vi "Prune to Directory.vi"(8 "error in (no error)":errorcluster, 11 "Path In":path) -> (0 "error out":errorcluster, 3 "Directory":path)   [LabVIEW 2021, in "File_CIF_U.lvlib"]
doc: "Check if file or directory. If file prune and return the directory."
uses:
  File_CIF_U.lvlib
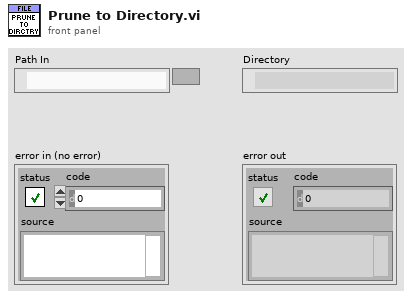
[diagram p1: front panel]
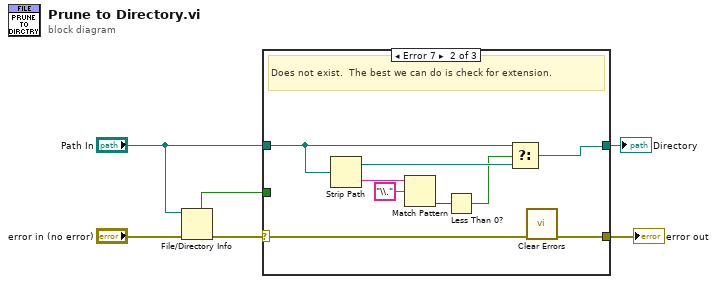
[diagram p0: block diagram]
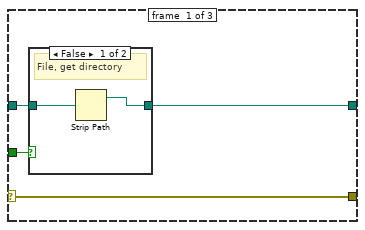
[diagram p2: hidden frame]
diagram:
  n1 = File/Directory Info(path="Path In", error in="error in (no error)") -> (directory=w6:bool, error out=w2:errorcluster)  [unwired: 5 out]
  n2 = case shown="Error 7" w2 {
    selector: w2 -> [w7 w15 w23]
    tunnel: w6 -> [w10 _ _]
    tunnel: [w9 w16 w24] -> w5
    tunnel: "Path In" -> [w8 w17 w24]
    tunnel: [w7 w14 w23] -> w1
    frame #0 {
      n3 = case shown="False" w10 {
        tunnel: w8 -> [w12 w13]
        tunnel: [w11 w13] -> w9
        frame False {
          # "File, get directory"
          n4 = Strip Path(path=w12) -> (stripped path=w11:path)  [unwired: 1 out]
        }
        frame True {
          # "Directory"
        }
      }
    }
    frame #1 {
      # "Does not exist.  The best we can do is check for extension."
      n5 = Strip Path(path=w17) -> (stripped path=w19:path, name=w22:string)
      n6 = Match Pattern(string=w22, regular expression="\\.") -> (offset past match=w20:i32)  [unwired: 1 in, 3 out]
      n7 = Less Than 0?(x=w20) -> (x < 0?=w18:bool)
      n8 = Select(t=w17, s=w18, f=w19) -> (s? t:f=w16:path)
      n9 = call <vilib>:"Clear Errors.vi"("error in (no error)"=w15) -> ("error out"=w14:errorcluster)  [unwired: 5 in, 1 out]
    }
    frame #2 {
    }
  }
  "Directory" <- w5
  "error out" <- w1
